vi "Test List States in Category.vi"(8 "error in (no error)":errorcluster) -> (0 "error out":errorcluster)   [LabVIEW 2013, in "TEST JKI State Machine API.lvlib"]
uses:
  TEST JKI State Machine API.lvlib
  <vilib>/addons/_JKI Toolkits/Caraya/classes/Assert/Assert.lvclass
  <vilib>/addons/_JKI Toolkits/Caraya/classes/Test/Test.lvclass
  source/JKI SM/JKI SM.lvclass
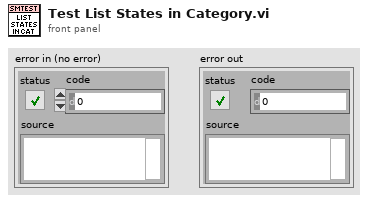
[diagram p1: front panel]
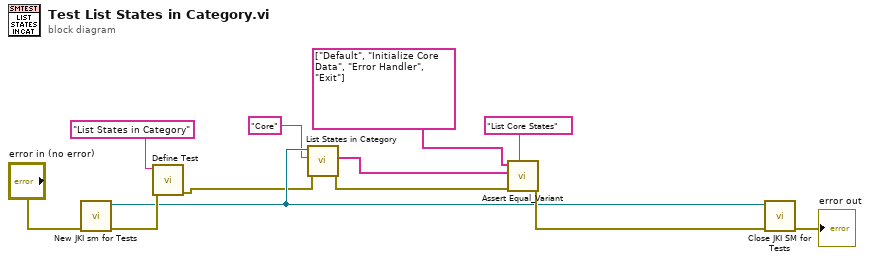
[diagram p0: block diagram]
diagram:
  n1 = call "New JKI sm for Tests.vi"("error in (no error)"="error in (no error)") -> ("error out"=w12:errorcluster, "JKI SM out"=w6:refnum<class "JKI SM.lvclass">)  [unwired: 9 in]
  n2 = call <vilib>:"Define Test.vi"("error in (no error)"=w12, "Label (VI Title)"="List States in Category") -> ("error out"=w2:errorcluster)  [unwired: 9 in]
  n3 = call "List States in Category.vi"("error in (no error)"=w2, "Category"="Core", "JKI SM in"=w6) -> ("error out"=w1:errorcluster, "States"=w4:string[])  [unwired: 4 in, 3 out]
  n4 = call <vilib>:"Assert Equal_Variant.vi"("Label"="List Core States", "error in (no error)"=w1, "Y"=w4, "X"=string[] ["Default", "Initialize Core Data", "Error Handler", "Exit"] ("States")) -> ("error out"=w9:errorcluster)  [unwired: 7 in]
  n5 = call "Close JKI SM for Tests.vi"("error in (no error)"=w9, "JKI SM in"=w6) -> ("error out"=→"error out":errorcluster)  [unwired: 9 in]
